vi "SMO.Dictionary.GetPublicEvents.vi"(8 "error in (no error)":errorcluster, 11 "SMO.Dictionary in":refnum<class "SMO.Dictionary.lvclass">) -> (0 "error out":errorcluster, 2 "Public Events":T1, 3 "SMO.Dictionary out":refnum<class "SMO.Dictionary.lvclass">)   [LabVIEW 2013, in "SMO.Dictionary.lvlib" / "SMO.Dictionary.lvclass"]
uses:
  SMO.Dictionary.lvclass
  Typedefs/PublicEvents--Cluster.ctl
  Typedefs/PrivateEvents--SMO.Dictionary.KeyValue-Pair.ctl
  SMO.Dictionary.lvclass/SMO.Dictionary.ctl
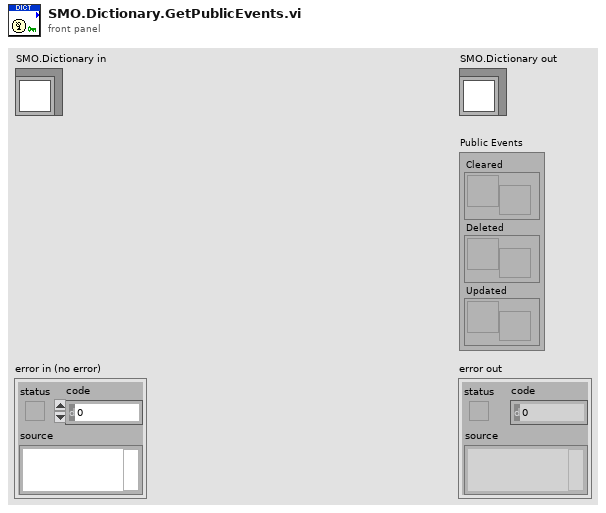
[diagram p1: front panel]
types:
  T1 = typedef "SMO.Dictionary.lvlib/SMO.Dictionary.lvclass/PublicEvents--Cluster.ctl" = cluster{"Cleared":refnum<user-event>, "Deleted":refnum<user-event>, "Updated":refnum<user-event>}
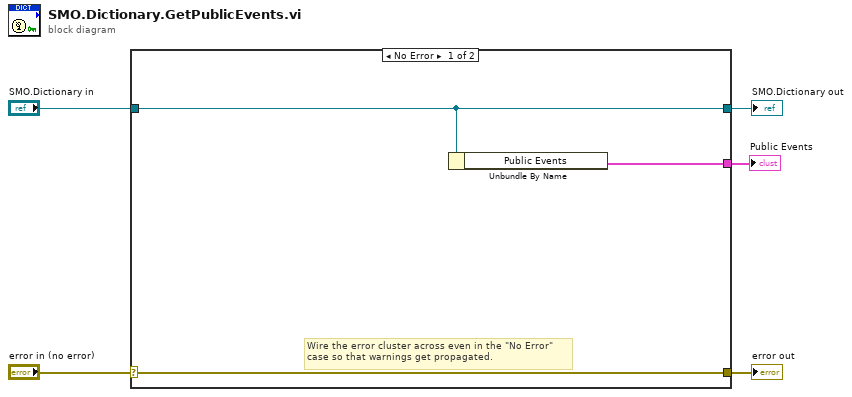
[diagram p0: block diagram]
diagram:
  n1 = case shown="No Error" "error in (no error)" {
    selector: "error in (no error)" -> [w8 w10]
    tunnel: [w8 w10] -> w4
    tunnel: [w7 w9] -> w2
    tunnel: "SMO.Dictionary in" -> [w7 w9]
    tunnel: [w6 _] -> w1
    frame No Error {
      # "Wire the error cluster across even in the \"No Error\"\ncase so that warnings get propagated."
      n2 = Unbundle By Name(w7) -> ("Public Events"=w6:T1)
    }
    frame Error {
    }
  }
  "error out" <- w4
  "SMO.Dictionary out" <- w2
  "Public Events" <- w1
